vi "Data_Write_Disk.vi"(8 "error in (no error)":errorcluster, 9 "wfm info":T2(array[cluster]) {"reserved2" format="%.2f"; "reserved1" format="%.2f"; "offset" format="%^.3e"; "gain" format="%^.3e"; "xIncrement" format="%^.3e"; "relativeInitialX" format="%^.3e"; "absoluteInitialX" format="%^.3e"}, 10 "dataset":i16[][](array[numeric]), 11 "QMH ICR Cluster":T1) -> (0 "error out":errorcluster, 1 "Mass Spectrum":cluster{sgl[], sgl[]}[](array[cluster]), 2 "Frequency Spectrum":cluster{sgl[], sgl[]}[](array[cluster]), 3 "Dataset Signal":cluster{sgl[], sgl[]}[](array[cluster]), 4 "Mass Accumulated":cluster{"mass":sgl[], sgl[]}[](array[cluster]))   [LabVIEW 2024]
doc: "This VI writes a dataset to disk, and process the corresponding frequency and mass spectra.\n- the dataset is first splitted into single acquisitions\n- one binary file and one XML file are written to disk for each acquisition\n- in case of several accumulations, the accumulated signal is updated\n- the frequency and mass spectra are processed, but not written to disk"
uses:
  controls/QMH_ICR_Cluster.ctl
  controls/HARDWARE_Resources.ctl
  controls/PROCESSING_Inputs.ctl
  controls/LOOPS_Inputs.ctl
  controls/OPO_Inputs.ctl
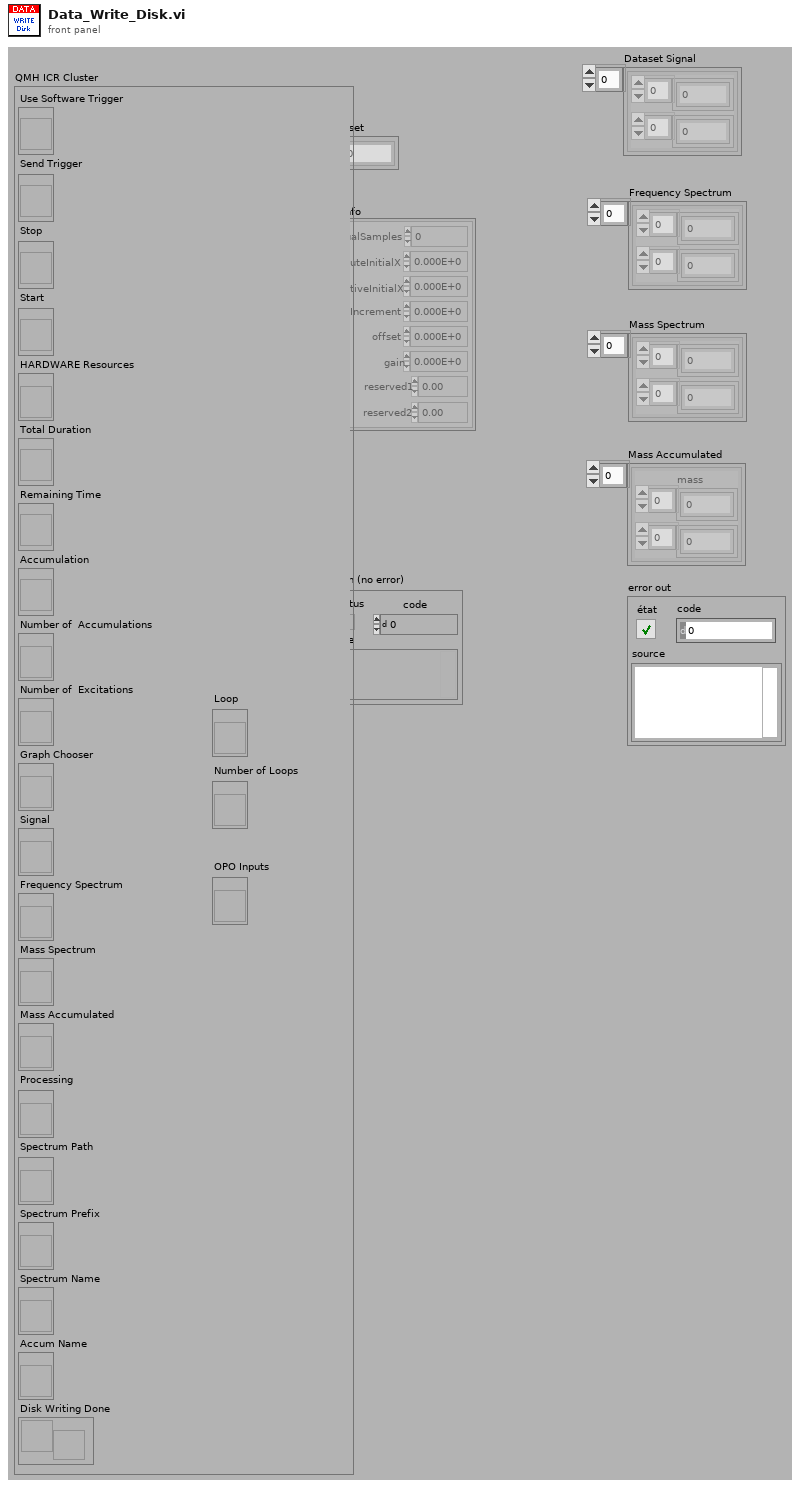
[diagram p1: front panel]
types:
  T1 = typedef "QMH_ICR_Cluster.ctl" = cluster{"Use Software Trigger":refnum<vi>, "Send Trigger":refnum<vi>, "Stop":refnum<vi>, "Start":refnum<vi>, "HARDWARE Resources":refnum<vi>, "Total Duration":refnum<vi>, "Remaining Time":refnum<vi>, "Accumulation":refnum<vi>, "Number of  Accumulations":refnum<vi>, "Number of  Excitations":refnum<vi>, "Graph Chooser":refnum<vi>, "Signal":refnum<vi>, "Frequency Spectrum":refnum<vi>, "Mass Spectrum":refnum<vi>, "Mass Accumulated":refnum<vi>, "Processing":refnum<vi>, "Spectrum Path":refnum<vi>, "Spectrum Prefix":refnum<vi>, "Spectrum Name":refnum<vi>, "Accum Name":refnum<vi>, "Disk Writing Done":refnum<notifier>, "Loop":refnum<vi>, "Number of Loops":refnum<vi>, "OPO Inputs":refnum<vi>}
  T2 = cluster{"actualSamples":i32, "absoluteInitialX":dbl, "relativeInitialX":dbl, "xIncrement":dbl, "offset":dbl, "gain":dbl, "reserved1":dbl, "reserved2":dbl}[]
  T3 = typedef "PROCESSING_Inputs.ctl" = cluster{"Reference Mass":dbl, "Cyclotron Freq":dbl, "Magnetron Freq":dbl}
  T4 = cluster{"actualSamples":i32, "absoluteInitialX":dbl, "relativeInitialX":dbl, "xIncrement":dbl, "offset":dbl, "gain":dbl, "reserved1":dbl, "reserved2":dbl}
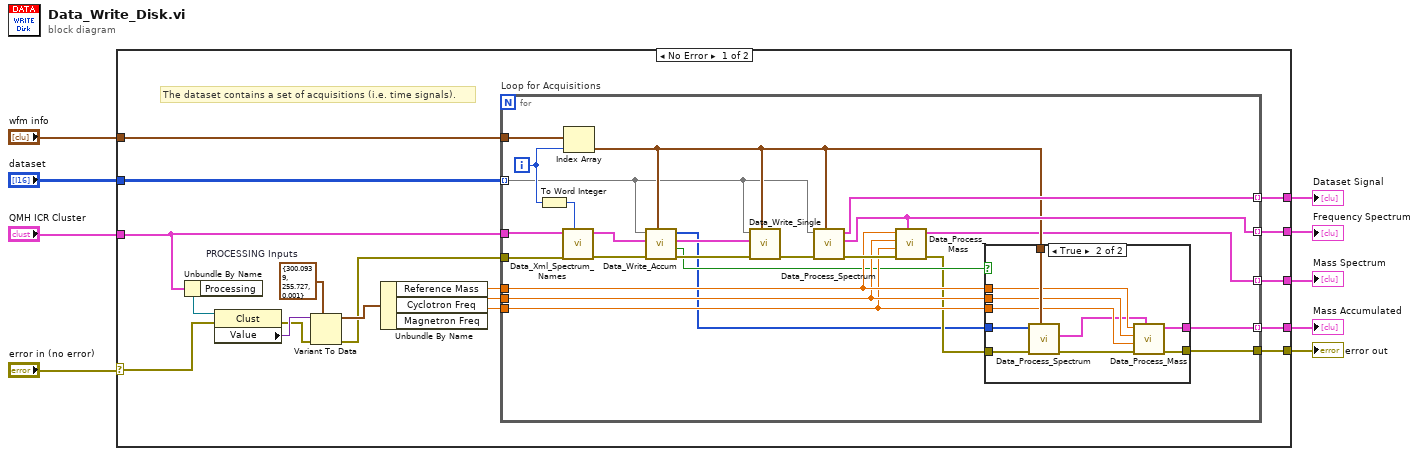
[diagram p0: block diagram]
diagram:
  n1 = case shown="No Error" "error in (no error)" {
    selector: "error in (no error)" -> [w15 w63]
    tunnel: [w13 w63] -> w5
    tunnel: "dataset" -> [w27 _]
    tunnel: [w26 _] -> w2
    tunnel: "QMH ICR Cluster" -> [w20 _]
    tunnel: "wfm info" -> [w25 _]
    tunnel: [w12 _] -> w1
    tunnel: [w11 _] -> w4
    tunnel: [w10 _] -> w3
    frame No Error {
      w17 = T3 {"Reference Mass"=300.0939, "Cyclotron Freq"=255.727, "Magnetron Freq"=0.001}  # PROCESSING Inputs
      # "The dataset contains a set of acquisitions (i.e. time signals)."
      n2 = Unbundle By Name(w20) -> ("Processing"=w24:refnum<vi>)
      n3 = property class="Clust"(reference=w24, error in=w15) -> (error out=w18:errorcluster, "Value"=w19:variant)  [unwired: 1 out]
      n4 = Variant To Data(error in=w18, type=w17, Variant=w19) -> (data=w16:T3, error out=w14:errorcluster)
      n5 = Unbundle By Name(w16) -> ("Reference Mass"=w23:dbl, "Cyclotron Freq"=w22:dbl, "Magnetron Freq"=w21:dbl)
      n6 = for "Loop for Acquisitions" {
        tunnel: w27 -> [w28] mode=indexing
        tunnel: [w51] -> w26 mode=indexing
        tunnel: w25 -> [w49]
        tunnel: w23 -> [w36]
        tunnel: w22 -> [w35]
        tunnel: w21 -> [w34]
        tunnel: w20 -> [w48]
        tunnel: w14 -> [w42]
        tunnel: [w38] -> w13
        tunnel: [w39] -> w12 mode=indexing
        tunnel: [w33] -> w11 mode=indexing
        tunnel: [w32] -> w10 mode=indexing
        i -> [w41]
        n7 = To Word Integer(number=w41) -> (16bit integer=w40:i16)
        n8 = call "Data_Xml_Spectrum_Names.vi"("Acquisition Number"=w40, "error in (no error)"=w42, "QMH ICR Cluster"=w48) -> ("error out"=w46:errorcluster, "QMH ICR Cluster"=w47:T1)  [unwired: 7 in]
        n9 = Index Array(array=w49, index=w41) -> (element=w37:T4)
        n10 = call "Data_Write_Accum.vi"("wfm info"=w37, "error in (no error)"=w46, "QMH ICR Cluster"=w47, "data"=w28) -> ("error out"=w45:errorcluster, "Is Accumulated ?"=w31:bool, "QMH ICR Cluster"=w44:T1, "data"=w29:i16[])  [unwired: 4 in]
        n11 = call "Data_Write_Single.vi"("wfm info"=w37, "error in (no error)"=w45, "QMH ICR Cluster"=w44, "data"=w28) -> ("error out"=w50:errorcluster)  [unwired: 6 in, 1 out]
        n12 = call "Data_Process_Spectrum.vi"("wfm info"=w37, "error in"=w50, "dataset"=w28) -> ("error out"=w43:errorcluster, "Frequency Spectrum"=w39:cluster{sgl[], sgl[]}, "Dataset Signal"=w51:cluster{sgl[], sgl[]})  [unwired: 6 in]
        n13 = call "Data_Process_Mass.vi"("Frequency Spectrum"=w39, "error in"=w43, "Mag. Frequency (kHz)"=w34, "Cycl. Frequency (kHz)"=w35, "Reference mass (u)"=w36) -> ("error out"=w30:errorcluster, "Mass Spectrum"=w33:cluster{"mass":sgl[], sgl[]})  [unwired: 5 in]
        n14 = case shown="True" w31 {
          tunnel: [w52 w62] -> w38
          tunnel: w37 -> [_ w61]
          tunnel: w36 -> [_ w60]
          tunnel: w35 -> [_ w59]
          tunnel: w34 -> [_ w58]
          tunnel: [_ w55] -> w32
          tunnel: w29 -> [_ w54]
          tunnel: w30 -> [w52 w53]
          frame False {
          }
          frame True {
            n15 = call "Data_Process_Spectrum.vi"("wfm info"=w61, "error in"=w53, "dataset"=w54) -> ("error out"=w56:errorcluster, "Frequency Spectrum"=w57:cluster{sgl[], sgl[]})  [unwired: 6 in, 1 out]
            n16 = call "Data_Process_Mass.vi"("Frequency Spectrum"=w57, "error in"=w56, "Mag. Frequency (kHz)"=w58, "Cycl. Frequency (kHz)"=w59, "Reference mass (u)"=w60) -> ("error out"=w62:errorcluster, "Mass Spectrum"=w55:cluster{"mass":sgl[], sgl[]})  [unwired: 5 in]
          }
        }
      }
    }
    frame Error {
    }
  }
  "error out" <- w5
  "Dataset Signal" <- w2
  "Frequency Spectrum" <- w1
  "Mass Spectrum" <- w4
  "Mass Accumulated" <- w3
